vi "Initialize.vi"(8 "error in":errorcluster, 10 "parameters":variant, 11 "voltage in":refnum<class "Voltage.lvclass">) -> (0 "error out":errorcluster, 2 "summary":T2[](array[typedef]), 3 "data value reference":T1)   [LabVIEW 2014, in "Voltage.lvclass"]
doc: "This Vi initializes the data of a node its default state.\nThe object is not created inside of this ViI, beacuase it is created from a File depending on user selection."
uses:
  Voltage.lvclass
  cRIO Repo/ChannelData.ctl
  cRIO Repo/cRIORepo.lvclass
  Channel/Channel.lvclass
  Configuration Framework/Node/NISE_CEF_Node.lvclass
  Configuration Framework/Node/Summary.ctl
  Configuration Framework/Node/NodeRef.ctl
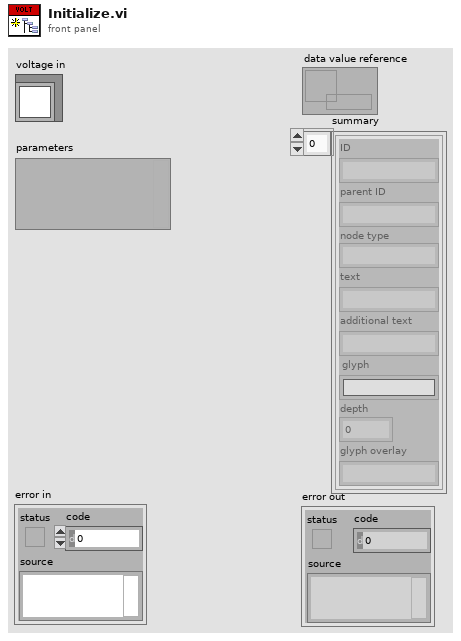
[diagram p1: front panel]
types:
  T1 = typedef "NISE_CEF_Node.lvclass/NodeRef.ctl" = refnum<data-value>
  T2 = typedef "NISE_CEF_Node.lvclass/Summary.ctl" = cluster{"ID":string, "parent ID":string, "node type":string, "text":string, "additional text":string, "glyph":string, "depth":i32, "glyph overlay":string}
  T3 = typedef "cRIORepo.lvclass/ChannelData.ctl" = cluster{"channel group":string, "channel name":string, "IO ":string, "sensor ID":string, "description":string, "system":string, "channel type":string}
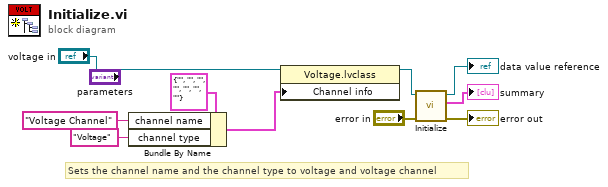
[diagram p0: block diagram]
diagram:
  # "Sets the channel name and the channel type to voltage and voltage channel"
  n1 = Bundle By Name(cluster=T3 {"channel group"="", "channel name"="", "IO "="", "sensor ID"="", "description"="", "system"="", "channel type"=""} ("channel info"), "channel name"="Voltage Channel" ("channel Name"), "channel type"="Voltage" ("channelType")) -> (w3:T3)
  n2 = property class="Voltage.lvclass"(reference="voltage in", "Channel info"=w3) -> (reference out=w5:refnum<class "Voltage.lvclass">)  [unwired: 1 in, 1 out]
  n3 = call-parent "Initialize.vi"("error in"="error in", "node in"=w5) -> ("error out"=→"error out":errorcluster, "summary"=→"summary":T2[], "data value reference"=→"data value reference":T1)  [unwired: 7 in]
